vi "SetGraphLegend1Graph.vi"(4 "error in (no error)":errorcluster, 6 "ConfigTotale":T2, 7 "ClusterRefGraphs":T1) -> (0 "error out":errorcluster)   [LabVIEW 2017]
uses:
  DefDeType/ConfigTotale.ctl
  DefDeType/VoltageChannels.ctl
  DefDeType/WBridgeChannels.ctl
  DefDeType/Configuration.ctl
panel:
  out "entier 32 bits non signé":u32
  out "appended array":string[](array[string])
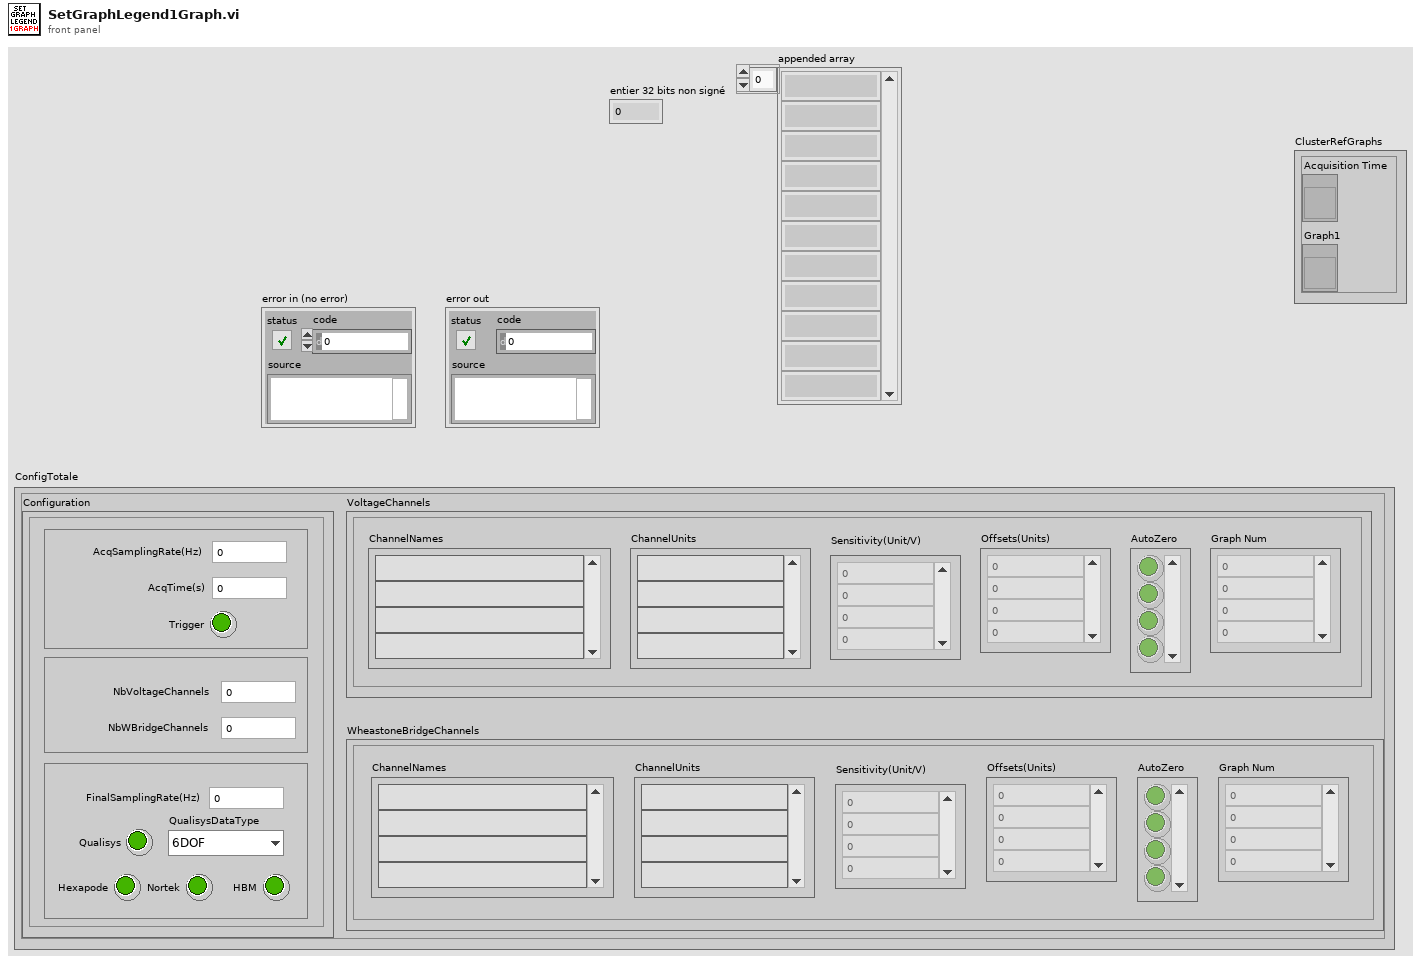
[diagram p1: front panel]
types:
  T1 = cluster{"Acquisition Time":refnum<vi>, "Graph1":refnum<vi>}
  T2 = typedef "ConfigTotale.ctl" = cluster{"VoltageChannels":T3, "WheastoneBridgeChannels":T4, "Configuration":T5}
  T3 = typedef "VoltageChannels.ctl" = cluster{"ChannelNames":string[], "Sensitivity(Unit/V)":dbl[], "AutoZero":bool[], "ChannelUnits":string[], "Offsets(Units)":dbl[], "Graph Num":u8[]}
  T4 = typedef "WBridgeChannels.ctl" = cluster{"ChannelNames":string[], "Sensitivity(Unit/V)":dbl[], "AutoZero":bool[], "ChannelUnits":string[], "Offsets(Units)":dbl[], "Graph Num":u8[]}
  T5 = typedef "Configuration.ctl" = cluster{"AcqSamplingRate(Hz)":u32, "AcqTime(s)":u32, "Trigger":bool, "NbVoltageChannels":u32, "NbWBridgeChannels":u32, "Qualisys":bool, "Hexapode":bool, "FinalSamplingRate(Hz)":u32, "QualisysDataType":enum16{"6DOF", "3DTracking", "6DOF + 3D"}, "Nortek":bool, "HBM":bool}
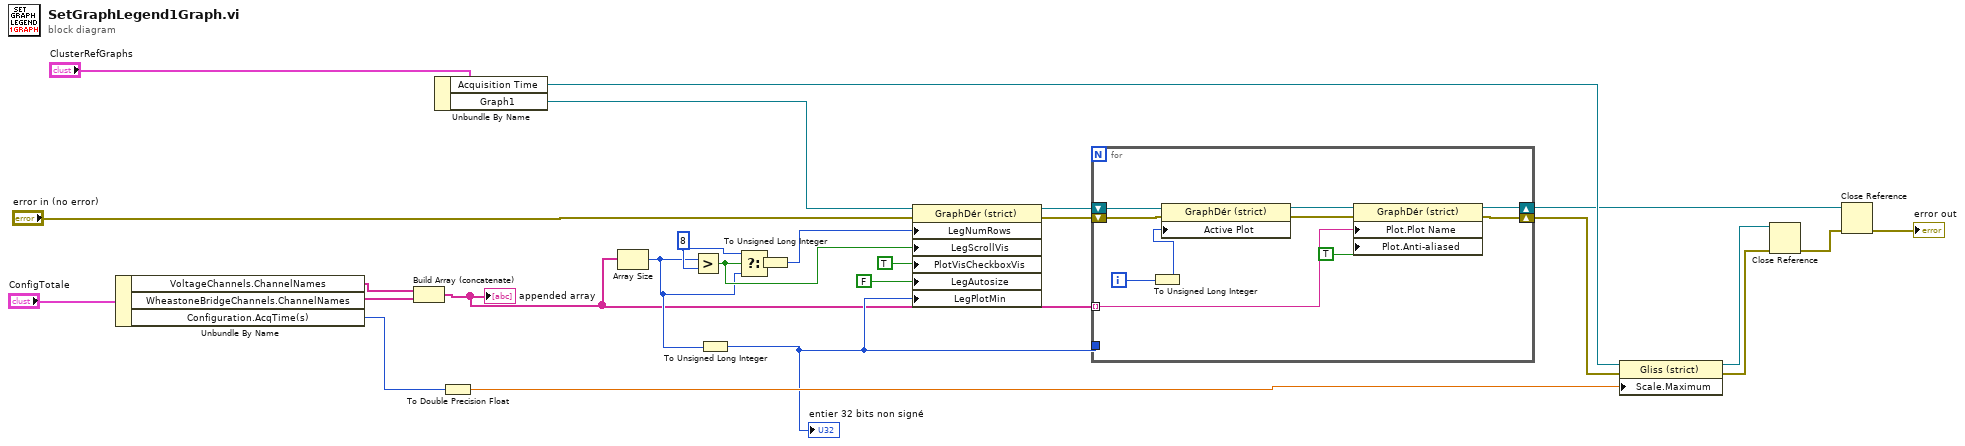
[diagram p0: block diagram]
diagram:
  w15 = 8 ("y")
  n1 = Unbundle By Name("ConfigTotale") -> ("VoltageChannels.ChannelNames"=w21:string[], "WheastoneBridgeChannels.ChannelNames"=w20:string[], "Configuration.AcqTime(s)"=w19:u32)
  n2 = Build Array (concatenate)(w21, w20) -> (w3:string[])
  "appended array" <- w3
  n3 = Unbundle By Name("ClusterRefGraphs") -> ("Acquisition Time"=w16:refnum<vi>, "Graph1"=w17:refnum<vi>)
  n4 = To Double Precision Float(number=w19) -> (double precision float=w26:dbl)
  n5 = Array Size(array=w3) -> (size(s)=w5:i32)
  n6 = Greater?(x=w5, y=w15) -> (0:w6:bool)
  n7 = To Unsigned Long Integer(number=w5) -> (unsigned 32bit integer=w4:u32)
  "entier 32 bits non signé" <- w4
  n8 = Select(t=w15, s=w6, f=w5) -> (s? t:f=w14:i32)
  n9 = To Unsigned Long Integer(number=w14) -> (unsigned 32bit integer=w7:u32)
  n10 = property class="GraphDér (strict)"(reference=w17, error in="error in (no error)", "LegNumRows"=w7, "LegScrollVis"=w6, "PlotVisCheckboxVis"=TRUE ("Légende:Case de visibilité du tracé visible"), "LegAutosize"=FALSE ("Légende:Redimensionnement automatique"), "LegPlotMin"=w4) -> (reference out=w24:refnum<vi>, error out=w23:errorcluster)
  n11 = for {
    shift-right: [w32] -> w2
    shift-left: w23 -> [w35]
    tunnel: w3 -> [w27] mode=indexing
    tunnel: w4 -> [_]
    shift-right: [w31] -> w8
    shift-left: w24 -> [w36]
    i -> [w29]
    n12 = To Unsigned Long Integer(number=w29) -> (unsigned 32bit integer=w30:u32)
    n13 = property class="GraphDér (strict)"(reference=w36, error in=w35, "Active Plot"=w30) -> (reference out=w33:refnum<vi>, error out=w34:errorcluster)
    n14 = property class="GraphDér (strict)"(reference=w33, error in=w34, "Plot.Plot Name"=w27, "Plot.Anti-aliased"=TRUE ("Tracé.Visible")) -> (reference out=w31:refnum<vi>, error out=w32:errorcluster)
  }
  n15 = property class="Gliss (strict)"(reference=w16, error in=w2, "Scale.Maximum"=w26) -> (reference out=w9:refnum<vi>, error out=w11:errorcluster)
  n16 = Close Reference(reference=w9, error in (no error)=w11) -> (error out=w1:errorcluster)
  n17 = Close Reference(reference=w8, error in (no error)=w1) -> (error out=→"error out":errorcluster)
